vi "PI_Start_Wave_Gen.vi"(0 "System no.":i32, 11 "error in":errorcluster, 12 "Axis":enum32{"x-y", "x-z", "y-z"}(ring)) -> (4 "System no. (dup)":i32, 15 "error out":errorcluster)   [LabVIEW 2009]
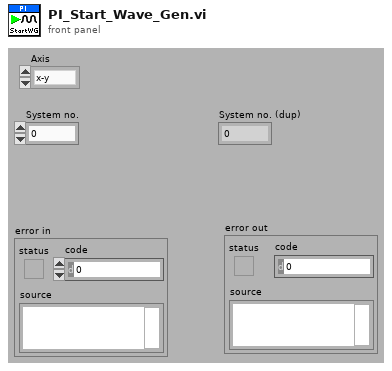
[diagram p1: front panel]
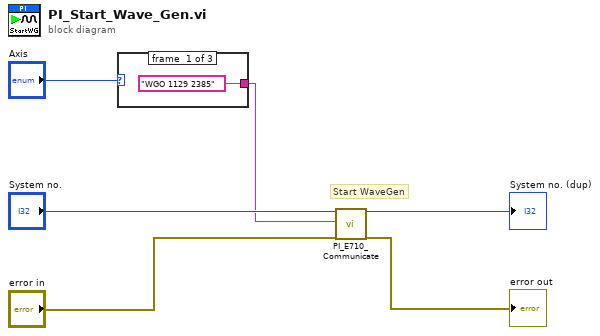
[diagram p0: block diagram]
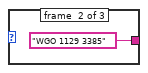
[diagram p2: hidden frame]
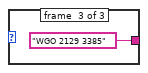
[diagram p3: hidden frame]
diagram:
  # "Start WaveGen"
  n1 = case shown="\"x-y\", Default" "Axis" {
    tunnel: ["WGO 1129 2385" ("String to send") "WGO 1129 3385" ("String to send") "WGO 2129 3385" ("String to send")] -> w1
    frame #0 {
    }
    frame #1 {
    }
    frame #2 {
    }
  }
  n2 = call "PI_E710_Communicate.vi"("System no."="System no.", "String to send"=w1, "error in"="error in") -> ("System no. (dup)"=→"System no. (dup)":i32, "error out"=→"error out":errorcluster)  [unwired: 14 in, 1 out]
